vi "Scene info analyzer.vi"(6 "Map Entity Object Position":T2(array[cluster]), 7 "Current Player ID":i32, 8 "Max Player ID":i32) -> (0 "Enemy on 8 directions":T3, 1 "Closest valid target":T1, 2 "Farther Bullets on 8 directions":T3, 3 "Closer Bullets on 8 directions":T3, 4 "Current Player HP":dbl, 5 "Object on 8 directions":T3)   [LabVIEW 2021]
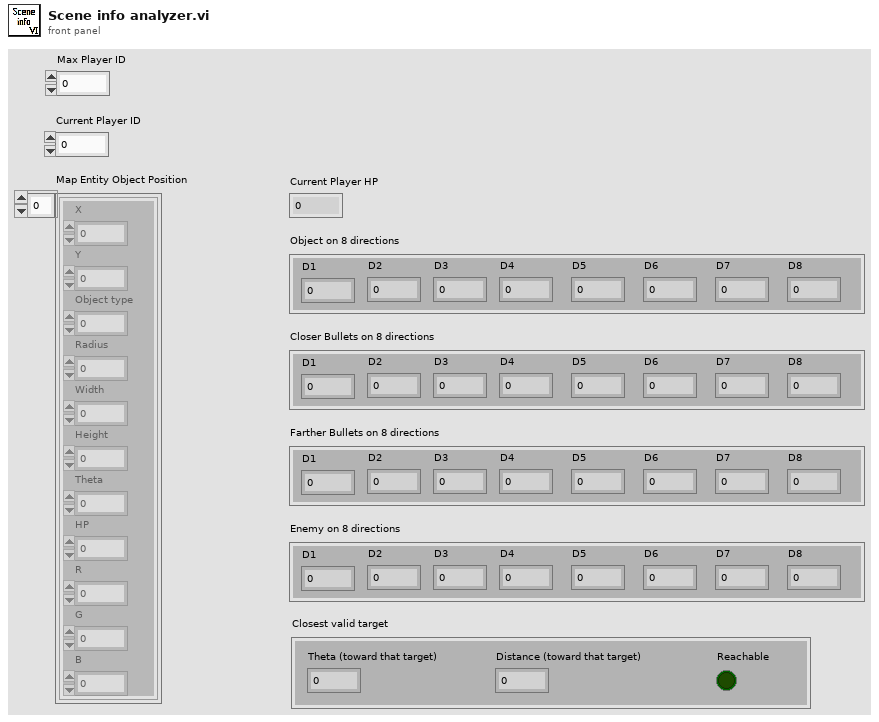
[diagram p1: front panel]
types:
  T1 = cluster{"Theta (toward that target)":dbl, "Distance (toward that target)":dbl, "Reachable":bool}
  T2 = cluster{"X":dbl, "Y":dbl, "Object type":dbl, "Radius":dbl, "Width":dbl, "Height":dbl, "Theta":dbl, "HP":dbl, "R":dbl, "G":dbl, "B":dbl}[]
  T3 = cluster{"D1":dbl, "D2":dbl, "D3":dbl, "D4":dbl, "D5":dbl, "D6":dbl, "D7":dbl, "D8":dbl}
  T4 = cluster{"X":dbl, "Y":dbl, "Object type":dbl, "Radius":dbl, "Width":dbl, "Height":dbl, "Theta":dbl, "HP":dbl, "R":dbl, "G":dbl, "B":dbl}
  T5 = cluster{"X":dbl, "Y":dbl, "Theta (toward that target)":dbl, "Theta (toward that target)":dbl, "Theta (toward that target)":dbl, "Theta (toward that target)":dbl}
  T6 = cluster{dbl, dbl, "Theta (toward that target)":dbl, "Theta (toward that target)":dbl, "Theta (toward that target)":dbl, "Theta (toward that target)":dbl}
  T7 = cluster{dbl, "D2":dbl, "D3":dbl, "D4":dbl, "D5":dbl, "D6":dbl, "D7":dbl, "D8":dbl}
  T8 = cluster{"D1":dbl, dbl, "D3":dbl, "D4":dbl, "D5":dbl, "D6":dbl, "D7":dbl, "D8":dbl}
  T9 = cluster{"D1":dbl, "D2":dbl, dbl, "D4":dbl, "D5":dbl, "D6":dbl, "D7":dbl, "D8":dbl}
  T10 = cluster{"D1":dbl, "D2":dbl, "D3":dbl, dbl, "D5":dbl, "D6":dbl, "D7":dbl, "D8":dbl}
  T11 = cluster{"D1":dbl, "D2":dbl, "D3":dbl, "D4":dbl, dbl, "D6":dbl, "D7":dbl, "D8":dbl}
  T12 = cluster{"D1":dbl, "D2":dbl, "D3":dbl, "D4":dbl, "D5":dbl, dbl, "D7":dbl, "D8":dbl}
  T13 = cluster{"D1":dbl, "D2":dbl, "D3":dbl, "D4":dbl, "D5":dbl, "D6":dbl, dbl, "D8":dbl}
  T14 = cluster{"D1":dbl, "D2":dbl, "D3":dbl, "D4":dbl, "D5":dbl, "D6":dbl, "D7":dbl, dbl}
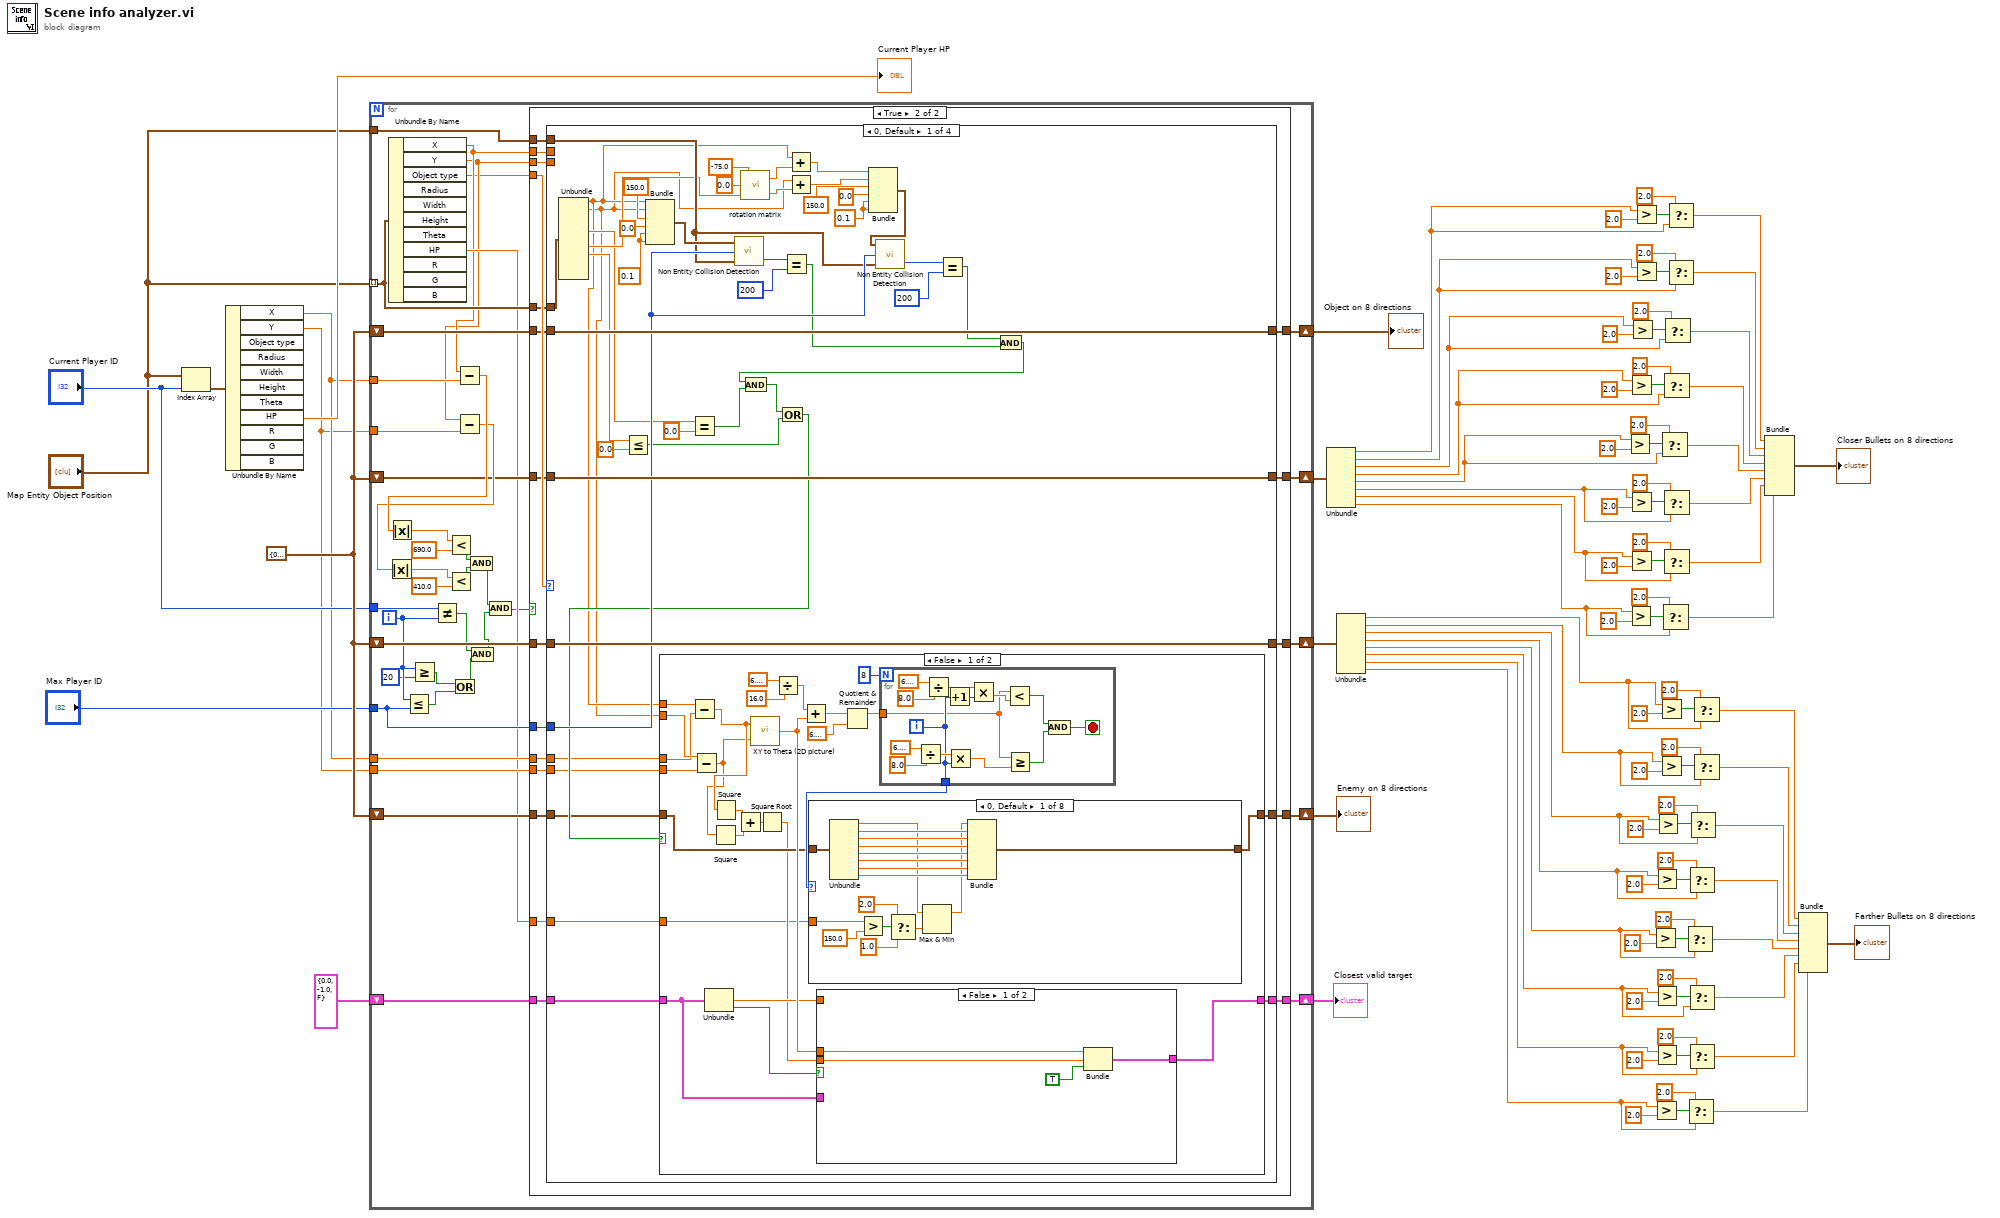
[diagram p0: block diagram]
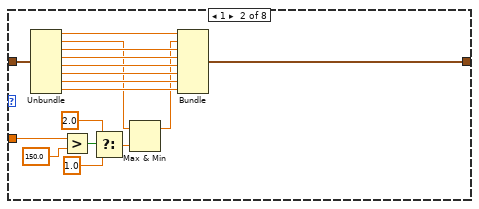
[diagram p3: hidden frame]
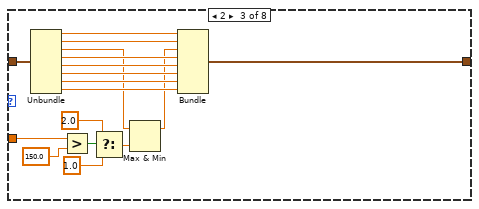
[diagram p4: hidden frame]
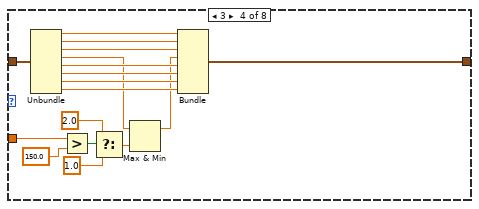
[diagram p5: hidden frame]
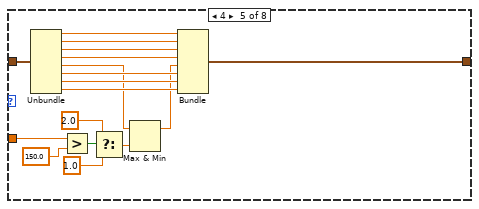
[diagram p6: hidden frame]
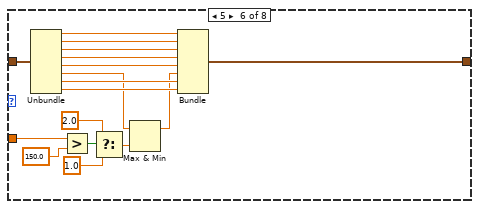
[diagram p7: hidden frame]
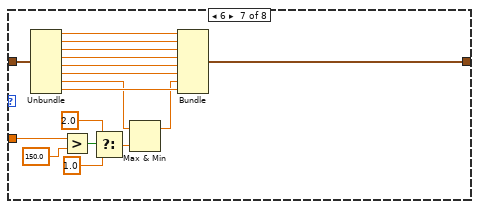
[diagram p8: hidden frame]
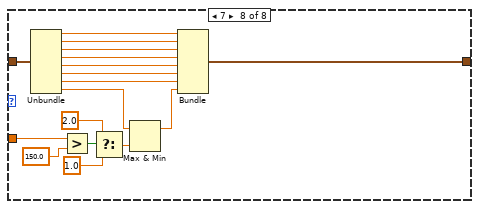
[diagram p9: hidden frame]
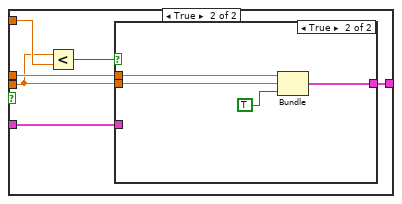
[diagram p10: hidden frame]
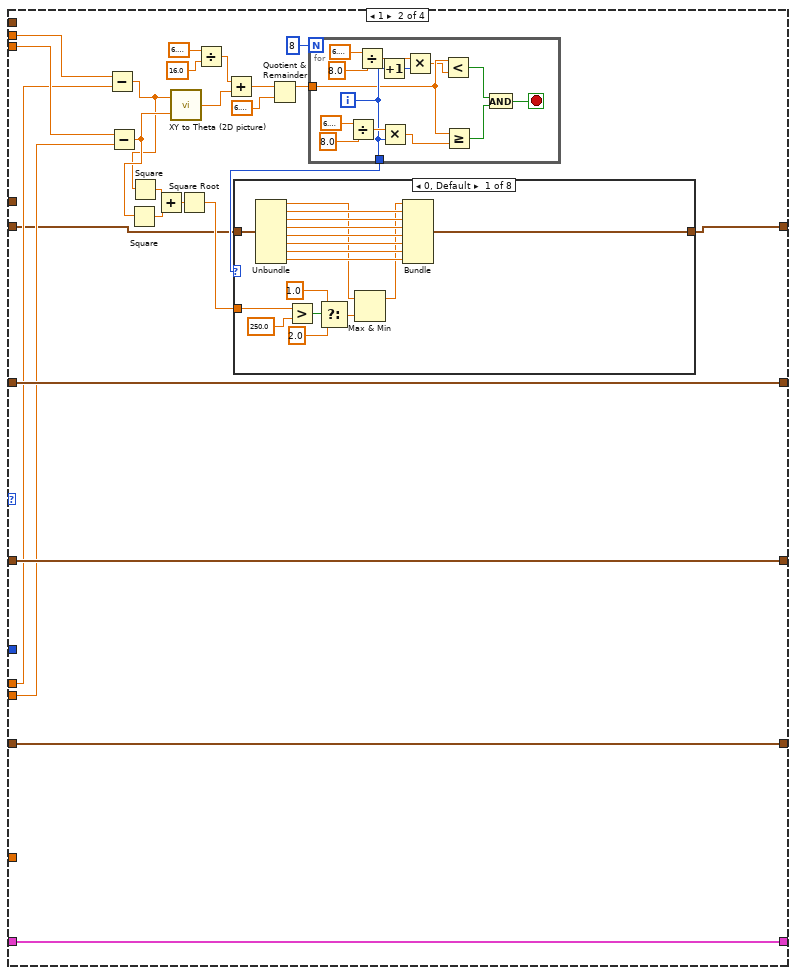
[diagram p13: hidden frame]
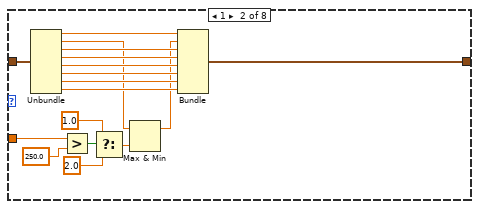
[diagram p14: hidden frame]
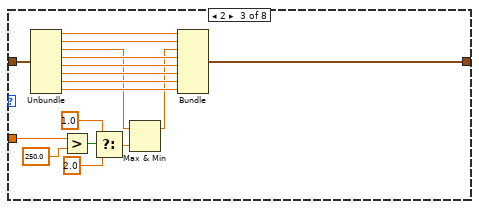
[diagram p15: hidden frame]
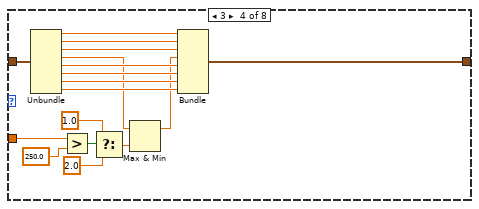
[diagram p16: hidden frame]
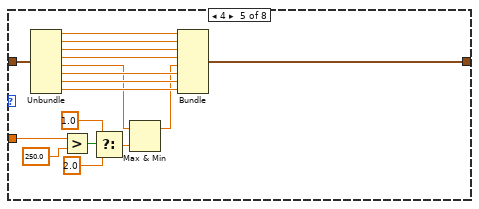
[diagram p17: hidden frame]
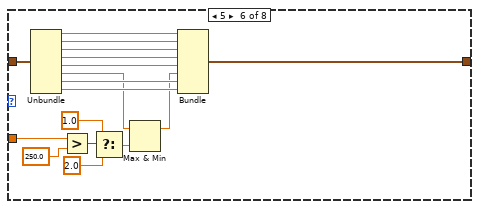
[diagram p18: hidden frame]
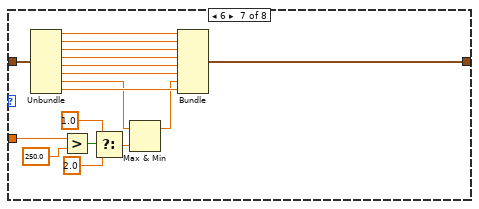
[diagram p19: hidden frame]
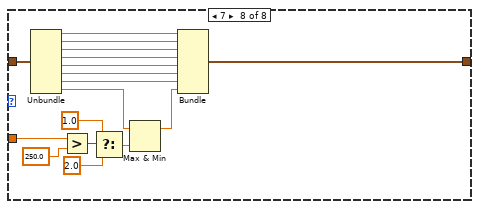
[diagram p20: hidden frame]
diagram:
  w93 = T3 {"D1"=0.0, "D2"=0.0, "D3"=0.0, "D4"=0.0, "D5"=0.0, "D6"=0.0, "D7"=0.0, "D8"=0.0} ("Object on 8 directions")
  n1 = Index Array(array="Map Entity Object Position", index="Current Player ID") -> (element=w96:T4)
  n2 = Unbundle By Name(w96) -> ("X"=w86:dbl, "Y"=w85:dbl, "HP"=→"Current Player HP":dbl)  [unwired: 8 out]
  n3 = for {
    shift-right: [w124] -> w94
    shift-left: w93 -> [w123]
    shift-right: [w122] -> w81
    shift-left: w93 -> [w121]
    shift-right: [w120] -> w80
    shift-left: w93 -> [w119]
    shift-right: [w117] -> w92
    shift-left: w93 -> [w118]
    tunnel: "Map Entity Object Position" -> [w110] mode=indexing
    tunnel: "Current Player ID" -> [w99]
    tunnel: w86 -> [w130]
    tunnel: w85 -> [w129]
    shift-right: [w115] -> w89
    shift-left: T1 {"Theta (toward that target)"=0.0, "Distance (toward that target)"=-1.0, "Reachable"=FALSE} ("Closest valid target") -> [w116]
    tunnel: "Max Player ID" -> [w108]
    tunnel: "Map Entity Object Position" -> [w109]
    tunnel: w86 -> [w107]
    tunnel: w85 -> [w106]
    i -> [w112]
    n4 = Unbundle By Name(w110) -> ("X"=w104:dbl, "Y"=w103:dbl, "Object type"=w98:dbl, "HP"=w105:dbl)  [unwired: 7 out]
    n5 = Less Or Equal?(x=w112, y=w108) -> (x <= y?=w114:bool)
    n6 = Greater Or Equal?(x=w112, y=20) -> (x >= y?=w113:bool)
    n7 = Not Equal?(x=w99, y=w112) -> (x != y?=w100:bool)
    n8 = Or(x=w113, y=w114) -> (x .or. y?=w102:bool)
    n9 = Subtract(x=w104, y=w130) -> (x-y=w126:dbl)
    n10 = Absolute Value(x=w126) -> (abs(x)=w128:dbl)
    n11 = Less?(x=w128, y=690.0) -> (x < y?=w134:bool)
    n12 = Subtract(x=w103, y=w129) -> (x-y=w125:dbl)
    n13 = Absolute Value(x=w125) -> (abs(x)=w127:dbl)
    n14 = Less?(x=w127, y=410.0) -> (x < y?=w133:bool)
    n15 = And(x=w134, y=w133) -> (x .and. y?=w135:bool)
    n16 = And(x=w100, y=w102) -> (x .and. y?=w101:bool)
    n17 = And(x=w135, y=w101) -> (x .and. y?=w97:bool)
    n18 = case shown="True" w97 {
      tunnel: [w140 w158] -> w124
      tunnel: w123 -> [w140 w157]
      tunnel: [w139 w156] -> w122
      tunnel: w121 -> [w139 w155]
      tunnel: [w138 w154] -> w120
      tunnel: w119 -> [w138 w153]
      tunnel: [w137 w149] -> w117
      tunnel: w118 -> [w137 w148]
      tunnel: [w136 w147] -> w115
      tunnel: w116 -> [w136 w146]
      tunnel: w98 -> [_ w159]
      tunnel: w110 -> [_ w152]
      tunnel: w109 -> [_ w151]
      tunnel: w108 -> [_ w150]
      tunnel: w107 -> [_ w145]
      tunnel: w106 -> [_ w144]
      tunnel: w105 -> [_ w143]
      tunnel: w104 -> [_ w142]
      tunnel: w103 -> [_ w141]
      frame False {
      }
      frame True {
        n19 = case shown="0, Default" w159 {
          tunnel: [w204 w398 w573 w752] -> w158
          tunnel: w157 -> [w204 w399 w574 w752]
          tunnel: [w203 w422 w597 w748] -> w156
          tunnel: w155 -> [w203 w422 w597 w751]
          tunnel: [w202 w421 w596 w749] -> w154
          tunnel: w153 -> [w202 w421 w596 w750]
          tunnel: w152 -> [w201 _ _ _]
          tunnel: w151 -> [w190 _ _ _]
          tunnel: w150 -> [w191 _ _ _]
          tunnel: [w173 w420 w595 w773] -> w149
          tunnel: w148 -> [w172 w420 w595 w773]
          tunnel: [w171 w419 w594 w772] -> w147
          tunnel: w146 -> [w170 w419 w594 w772]
          tunnel: w145 -> [w166 w401 w576 w754]
          tunnel: w144 -> [w165 w400 w575 w753]
          tunnel: w143 -> [w164 _ _ _]
          tunnel: w142 -> [_ w403 w578 w756]
          tunnel: w141 -> [_ w402 w577 w755]
          frame 0, Default {
            w193 = 0.1 ("Theta (toward that target)")
            w198 = 0.1 ("Theta (toward that target)")
            n20 = Unbundle(w201) -> ("X"=w168:dbl, "Y"=w167:dbl, "Width"=w177:dbl, "Theta"=w187:dbl, "HP"=w179:dbl)  [unwired: 6 out]
            n21 = Less Or Equal?(x=w179, y=0.0) -> (x <= y?=w169:bool)
            n22 = Bundle("X"=w168, "Y"=w167, "Theta (toward that target)"=150.0, "Theta (toward that target)"=0.0, "Theta (toward that target)"=w198, "Theta (toward that target)"=w198) -> (w197:T5)  [unwired: 1 in]
            n23 = Equal?(x=w177, y=0.0) -> (x = y?=w160:bool)
            n24 = call "Non Entity Collision Detection.vi"("Map Entity Objects Positions"=w190, "Max Player ID number"=w191, "Moving Object"=w197) -> ("Bullet hit Player No."=w196:i32)  [unwired: 1 out]
            n25 = call "rotation matrix.vi"("angle"=w187, "y"=0.0, "x"=-75.0) -> ("new y"=w180:dbl, "new x"=w181:dbl)
            n26 = Equal?(x=w196, y=200) -> (x = y?=w161:bool)
            n27 = Add(x=w168, y=w181) -> (x+y=w182:dbl)
            n28 = Add(x=w167, y=w180) -> (x+y=w183:dbl)
            n29 = Bundle(w182, w183, "Theta (toward that target)"=150.0, "Theta (toward that target)"=0.0, "Theta (toward that target)"=w193, "Theta (toward that target)"=w193) -> (w184:T6)  [unwired: 1 in]
            n30 = call "Non Entity Collision Detection.vi"("Map Entity Objects Positions"=w190, "Max Player ID number"=w191, "Moving Object"=w184) -> ("Bullet hit Player No."=w185:i32)  [unwired: 1 out]
            n31 = Equal?(x=w185, y=200) -> (x = y?=w162:bool)
            n32 = And(x=w162, y=w161) -> (x .and. y?=w163:bool)
            n33 = And(x=w163, y=w160) -> (x .and. y?=w175:bool)
            n34 = Or(x=w175, y=w169) -> (x .or. y?=w174:bool)
            n35 = case shown="False" w174 {
              tunnel: [w207 w397] -> w173
              tunnel: w172 -> [w208 w397]
              tunnel: [w218 w396] -> w171
              tunnel: w170 -> [w210 w396]
              tunnel: w168 -> [w230 _]
              tunnel: w167 -> [w229 _]
              tunnel: w166 -> [w227 _]
              tunnel: w165 -> [w228 _]
              tunnel: w164 -> [w205 _]
              frame False {
                n36 = Subtract(x=w230, y=w227) -> (x-y=w213:dbl)
                n37 = Subtract(x=w229, y=w228) -> (x-y=w212:dbl)
                n38 = Unbundle(w210) -> ("Distance (toward that target)"=w211:dbl, "Reachable"=w219:bool)  [unwired: 1 out]
                n39 = Square(x=w212) -> (x^2=w215:dbl)
                n40 = Square(x=w213) -> (x^2=w216:dbl)
                n41 = Add(x=w216, y=w215) -> (x+y=w214:dbl)
                n42 = call "XY to Theta (2D picture).vi"("y"=w212, "x"=w213) -> ("Theta"=w217:dbl)
                n43 = Square Root(x=w214) -> (sqrt(x)=w206:dbl)
                n44 = Divide(x=6.283185307179586, y=16.0) -> (x/y=w224:dbl)
                n45 = Add(x=w224, y=w217) -> (x+y=w223:dbl)
                n46 = case shown="False" w219 {
                  tunnel: [w369 w374] -> w218
                  tunnel: w217 -> [w368 w372]
                  tunnel: w206 -> [w367 w371]
                  tunnel: w211 -> [_ w376]
                  tunnel: w210 -> [_ w373]
                  frame False {
                    n47 = Bundle("Theta"=w368, w367, "Reachable"=TRUE) -> (w369:cluster{"Theta":dbl, dbl, "Reachable":bool})  [unwired: 1 in]
                  }
                  frame True {
                    n48 = Less?(x=w371, y=w376) -> (x < y?=w375:bool)
                    n49 = case shown="True" w375 {
                      tunnel: [w377 w380] -> w374
                      tunnel: w373 -> [w377 _]
                      tunnel: w372 -> [_ w379]
                      tunnel: w371 -> [_ w378]
                      frame False {
                      }
                      frame True {
                        n50 = Bundle("Theta"=w379, w378, "Reachable"=TRUE) -> (w380:cluster{"Theta":dbl, dbl, "Reachable":bool})  [unwired: 1 in]
                      }
                    }
                  }
                }
                n51 = Quotient & Remainder(x=w223, y=6.283185307179586) -> (x-y*floor(x/y)=w221:dbl)  [unwired: 1 out]
                n52 = for {
                  N: 8 -> [_]
                  tunnel: w221 -> [w383]
                  tunnel: [w385] -> w209
                  i -> [w385]
                  stop <- w386 stop-if-true
                  n53 = Divide(x=6.283185307179586, y=8.0) -> (x/y=w393:dbl)
                  n54 = Divide(x=6.283185307179586, y=8.0) -> (x/y=w390:dbl)
                  n55 = Increment(x=w385) -> (x+1=w389:i32)
                  n56 = Multiply(x=w393, y=w385) -> (x*y=w382:dbl)
                  n57 = Multiply(x=w390, y=w389) -> (x*y=w384:dbl)
                  n58 = Less?(x=w383, y=w384) -> (x < y?=w388:bool)
                  n59 = Greater Or Equal?(x=w383, y=w382) -> (x >= y?=w387:bool)
                  n60 = And(x=w388, y=w387) -> (x .and. y?=w386:bool)
                }
                n61 = case shown="0, Default" w209 {
                  tunnel: w208 -> [w247 w264 w281 w298 w315 w332 w349 w366]
                  tunnel: [w231 w251 w269 w287 w305 w323 w341 w359] -> w207
                  tunnel: w205 -> [w237 w255 w273 w291 w309 w327 w345 w363]
                  frame 0, Default {
                    n62 = Unbundle(w247) -> ("D1"=w233:dbl, "D2"=w244:dbl, "D3"=w243:dbl, "D4"=w242:dbl, "D5"=w241:dbl, "D6"=w240:dbl, "D7"=w239:dbl, "D8"=w238:dbl)
                    n63 = Greater?(x=w237, y=150.0) -> (0:w246:bool)
                    n64 = Select(t=2.0, s=w246, f=1.0) -> (s? t:f=w234:dbl)
                    n65 = Max & Min(x=w233, y=w234) -> (max(x,y)=w232:dbl)  [unwired: 1 out]
                    n66 = Bundle(w232, "D2"=w244, "D3"=w243, "D4"=w242, "D5"=w241, "D6"=w240, "D7"=w239, "D8"=w238) -> (w231:T7)  [unwired: 1 in]
                  }
                  frame 1 {
                    n67 = Unbundle(w264) -> ("D1"=w250:dbl, "D2"=w249:dbl, "D3"=w261:dbl, "D4"=w260:dbl, "D5"=w259:dbl, "D6"=w258:dbl, "D7"=w257:dbl, "D8"=w256:dbl)
                    n68 = Greater?(x=w255, y=150.0) -> (0:w263:bool)
                    n69 = Select(t=2.0, s=w263, f=1.0) -> (s? t:f=w252:dbl)
                    n70 = Max & Min(x=w249, y=w252) -> (max(x,y)=w248:dbl)  [unwired: 1 out]
                    n71 = Bundle("D1"=w250, w248, "D3"=w261, "D4"=w260, "D5"=w259, "D6"=w258, "D7"=w257, "D8"=w256) -> (w251:T8)  [unwired: 1 in]
                  }
                  frame 2 {
                    n72 = Unbundle(w281) -> ("D1"=w268:dbl, "D2"=w267:dbl, "D3"=w266:dbl, "D4"=w278:dbl, "D5"=w277:dbl, "D6"=w276:dbl, "D7"=w275:dbl, "D8"=w274:dbl)
                    n73 = Greater?(x=w273, y=150.0) -> (0:w280:bool)
                    n74 = Select(t=2.0, s=w280, f=1.0) -> (s? t:f=w270:dbl)
                    n75 = Max & Min(x=w266, y=w270) -> (max(x,y)=w265:dbl)  [unwired: 1 out]
                    n76 = Bundle("D1"=w268, "D2"=w267, w265, "D4"=w278, "D5"=w277, "D6"=w276, "D7"=w275, "D8"=w274) -> (w269:T9)  [unwired: 1 in]
                  }
                  frame 3 {
                    n77 = Unbundle(w298) -> ("D1"=w286:dbl, "D2"=w285:dbl, "D3"=w284:dbl, "D4"=w283:dbl, "D5"=w295:dbl, "D6"=w294:dbl, "D7"=w293:dbl, "D8"=w292:dbl)
                    n78 = Greater?(x=w291, y=150.0) -> (0:w297:bool)
                    n79 = Select(t=2.0, s=w297, f=1.0) -> (s? t:f=w288:dbl)
                    n80 = Max & Min(x=w283, y=w288) -> (max(x,y)=w282:dbl)  [unwired: 1 out]
                    n81 = Bundle("D1"=w286, "D2"=w285, "D3"=w284, w282, "D5"=w295, "D6"=w294, "D7"=w293, "D8"=w292) -> (w287:T10)  [unwired: 1 in]
                  }
                  frame 4 {
                    n82 = Unbundle(w315) -> ("D1"=w304:dbl, "D2"=w303:dbl, "D3"=w302:dbl, "D4"=w299:dbl, "D5"=w301:dbl, "D6"=w312:dbl, "D7"=w311:dbl, "D8"=w310:dbl)
                    n83 = Greater?(x=w309, y=150.0) -> (0:w314:bool)
                    n84 = Select(t=2.0, s=w314, f=1.0) -> (s? t:f=w306:dbl)
                    n85 = Max & Min(x=w301, y=w306) -> (max(x,y)=w300:dbl)  [unwired: 1 out]
                    n86 = Bundle("D1"=w304, "D2"=w303, "D3"=w302, "D4"=w299, w300, "D6"=w312, "D7"=w311, "D8"=w310) -> (w305:T11)  [unwired: 1 in]
                  }
                  frame 5 {
                    n87 = Unbundle(w332) -> ("D1"=w322:dbl, "D2"=w321:dbl, "D3"=w320:dbl, "D4"=w319:dbl, "D5"=w318:dbl, "D6"=w317:dbl, "D7"=w329:dbl, "D8"=w328:dbl)
                    n88 = Greater?(x=w327, y=150.0) -> (0:w331:bool)
                    n89 = Select(t=2.0, s=w331, f=1.0) -> (s? t:f=w324:dbl)
                    n90 = Max & Min(x=w317, y=w324) -> (max(x,y)=w316:dbl)  [unwired: 1 out]
                    n91 = Bundle("D1"=w322, "D2"=w321, "D3"=w320, "D4"=w319, "D5"=w318, w316, "D7"=w329, "D8"=w328) -> (w323:T12)  [unwired: 1 in]
                  }
                  frame 6 {
                    n92 = Unbundle(w349) -> ("D1"=w340:dbl, "D2"=w339:dbl, "D3"=w338:dbl, "D4"=w337:dbl, "D5"=w336:dbl, "D6"=w333:dbl, "D7"=w335:dbl, "D8"=w346:dbl)
                    n93 = Greater?(x=w345, y=150.0) -> (0:w348:bool)
                    n94 = Select(t=2.0, s=w348, f=1.0) -> (s? t:f=w342:dbl)
                    n95 = Max & Min(x=w335, y=w342) -> (max(x,y)=w334:dbl)  [unwired: 1 out]
                    n96 = Bundle("D1"=w340, "D2"=w339, "D3"=w338, "D4"=w337, "D5"=w336, "D6"=w333, w334, "D8"=w346) -> (w341:T13)  [unwired: 1 in]
                  }
                  frame 7 {
                    n97 = Unbundle(w366) -> ("D1"=w358:dbl, "D2"=w357:dbl, "D3"=w356:dbl, "D4"=w355:dbl, "D5"=w354:dbl, "D6"=w353:dbl, "D7"=w352:dbl, "D8"=w351:dbl)
                    n98 = Greater?(x=w363, y=150.0) -> (0:w365:bool)
                    n99 = Select(t=2.0, s=w365, f=1.0) -> (s? t:f=w360:dbl)
                    n100 = Max & Min(x=w351, y=w360) -> (max(x,y)=w350:dbl)  [unwired: 1 out]
                    n101 = Bundle("D1"=w358, "D2"=w357, "D3"=w356, "D4"=w355, "D5"=w354, "D6"=w353, "D7"=w352, w350) -> (w359:T14)  [unwired: 1 in]
                  }
                }
              }
              frame True {
              }
            }
          }
          frame 1 {
            n102 = Subtract(x=w403, y=w401) -> (x-y=w415:dbl)
            n103 = Subtract(x=w402, y=w400) -> (x-y=w416:dbl)
            n104 = Square(x=w416) -> (x^2=w413:dbl)
            n105 = Square(x=w415) -> (x^2=w412:dbl)
            n106 = Add(x=w412, y=w413) -> (x+y=w414:dbl)
            n107 = call "XY to Theta (2D picture).vi"("y"=w416, "x"=w415) -> ("Theta"=w411:dbl)
            n108 = Square Root(x=w414) -> (sqrt(x)=w418:dbl)
            n109 = Divide(x=6.283185307179586, y=16.0) -> (x/y=w408:dbl)
            n110 = Add(x=w408, y=w411) -> (x+y=w409:dbl)
            n111 = Quotient & Remainder(x=w409, y=6.283185307179586) -> (x-y*floor(x/y)=w410:dbl)  [unwired: 1 out]
            n112 = for {
              N: 8 -> [_]
              tunnel: w410 -> [w561]
              tunnel: [w562] -> w417
              i -> [w562]
              stop <- w563 stop-if-true
              n113 = Divide(x=6.283185307179586, y=8.0) -> (x/y=w570:dbl)
              n114 = Divide(x=6.283185307179586, y=8.0) -> (x/y=w567:dbl)
              n115 = Increment(x=w562) -> (x+1=w566:i32)
              n116 = Multiply(x=w570, y=w562) -> (x*y=w559:dbl)
              n117 = Multiply(x=w567, y=w566) -> (x*y=w560:dbl)
              n118 = Less?(x=w561, y=w560) -> (x < y?=w565:bool)
              n119 = Greater Or Equal?(x=w561, y=w559) -> (x >= y?=w564:bool)
              n120 = And(x=w565, y=w564) -> (x .and. y?=w563:bool)
            }
            n121 = case shown="0, Default" w417 {
              tunnel: w399 -> [w439 w456 w473 w490 w507 w524 w541 w558]
              tunnel: [w423 w443 w461 w479 w497 w515 w533 w551] -> w398
              tunnel: w418 -> [w429 w447 w465 w483 w501 w519 w537 w555]
              frame 0, Default {
                n122 = Unbundle(w439) -> ("D1"=w425:dbl, "D2"=w436:dbl, "D3"=w435:dbl, "D4"=w434:dbl, "D5"=w433:dbl, "D6"=w432:dbl, "D7"=w431:dbl, "D8"=w430:dbl)
                n123 = Greater?(x=w429, y=250.0) -> (0:w438:bool)
                n124 = Select(t=1.0, s=w438, f=2.0) -> (s? t:f=w426:dbl)
                n125 = Max & Min(x=w425, y=w426) -> (max(x,y)=w424:dbl)  [unwired: 1 out]
                n126 = Bundle(w424, "D2"=w436, "D3"=w435, "D4"=w434, "D5"=w433, "D6"=w432, "D7"=w431, "D8"=w430) -> (w423:T7)  [unwired: 1 in]
              }
              frame 1 {
                n127 = Unbundle(w456) -> ("D1"=w442:dbl, "D2"=w441:dbl, "D3"=w453:dbl, "D4"=w452:dbl, "D5"=w451:dbl, "D6"=w450:dbl, "D7"=w449:dbl, "D8"=w448:dbl)
                n128 = Greater?(x=w447, y=250.0) -> (0:w455:bool)
                n129 = Select(t=1.0, s=w455, f=2.0) -> (s? t:f=w444:dbl)
                n130 = Max & Min(x=w441, y=w444) -> (max(x,y)=w440:dbl)  [unwired: 1 out]
                n131 = Bundle("D1"=w442, w440, "D3"=w453, "D4"=w452, "D5"=w451, "D6"=w450, "D7"=w449, "D8"=w448) -> (w443:T8)  [unwired: 1 in]
              }
              frame 2 {
                n132 = Unbundle(w473) -> ("D1"=w460:dbl, "D2"=w459:dbl, "D3"=w458:dbl, "D4"=w470:dbl, "D5"=w469:dbl, "D6"=w468:dbl, "D7"=w467:dbl, "D8"=w466:dbl)
                n133 = Greater?(x=w465, y=250.0) -> (0:w472:bool)
                n134 = Select(t=1.0, s=w472, f=2.0) -> (s? t:f=w462:dbl)
                n135 = Max & Min(x=w458, y=w462) -> (max(x,y)=w457:dbl)  [unwired: 1 out]
                n136 = Bundle("D1"=w460, "D2"=w459, w457, "D4"=w470, "D5"=w469, "D6"=w468, "D7"=w467, "D8"=w466) -> (w461:T9)  [unwired: 1 in]
              }
              frame 3 {
                n137 = Unbundle(w490) -> ("D1"=w478:dbl, "D2"=w477:dbl, "D3"=w476:dbl, "D4"=w475:dbl, "D5"=w487:dbl, "D6"=w486:dbl, "D7"=w485:dbl, "D8"=w484:dbl)
                n138 = Greater?(x=w483, y=250.0) -> (0:w489:bool)
                n139 = Select(t=1.0, s=w489, f=2.0) -> (s? t:f=w480:dbl)
                n140 = Max & Min(x=w475, y=w480) -> (max(x,y)=w474:dbl)  [unwired: 1 out]
                n141 = Bundle("D1"=w478, "D2"=w477, "D3"=w476, w474, "D5"=w487, "D6"=w486, "D7"=w485, "D8"=w484) -> (w479:T10)  [unwired: 1 in]
              }
              frame 4 {
                n142 = Unbundle(w507) -> ("D1"=w496:dbl, "D2"=w495:dbl, "D3"=w494:dbl, "D4"=w491:dbl, "D5"=w493:dbl, "D6"=w504:dbl, "D7"=w503:dbl, "D8"=w502:dbl)
                n143 = Greater?(x=w501, y=250.0) -> (0:w506:bool)
                n144 = Select(t=1.0, s=w506, f=2.0) -> (s? t:f=w498:dbl)
                n145 = Max & Min(x=w493, y=w498) -> (max(x,y)=w492:dbl)  [unwired: 1 out]
                n146 = Bundle("D1"=w496, "D2"=w495, "D3"=w494, "D4"=w491, w492, "D6"=w504, "D7"=w503, "D8"=w502) -> (w497:T11)  [unwired: 1 in]
              }
              frame 5 {
                n147 = Unbundle(w524) -> ("D1"=w514:dbl, "D2"=w513:dbl, "D3"=w512:dbl, "D4"=w511:dbl, "D5"=w510:dbl, "D6"=w509:dbl, "D7"=w521:dbl, "D8"=w520:dbl)
                n148 = Greater?(x=w519, y=250.0) -> (0:w523:bool)
                n149 = Select(t=1.0, s=w523, f=2.0) -> (s? t:f=w516:dbl)
                n150 = Max & Min(x=w509, y=w516) -> (max(x,y)=w508:dbl)  [unwired: 1 out]
                n151 = Bundle("D1"=w514, "D2"=w513, "D3"=w512, "D4"=w511, "D5"=w510, w508, "D7"=w521, "D8"=w520) -> (w515:T12)  [unwired: 1 in]
              }
              frame 6 {
                n152 = Unbundle(w541) -> ("D1"=w532:dbl, "D2"=w531:dbl, "D3"=w530:dbl, "D4"=w529:dbl, "D5"=w528:dbl, "D6"=w525:dbl, "D7"=w527:dbl, "D8"=w538:dbl)
                n153 = Greater?(x=w537, y=250.0) -> (0:w540:bool)
                n154 = Select(t=1.0, s=w540, f=2.0) -> (s? t:f=w534:dbl)
                n155 = Max & Min(x=w527, y=w534) -> (max(x,y)=w526:dbl)  [unwired: 1 out]
                n156 = Bundle("D1"=w532, "D2"=w531, "D3"=w530, "D4"=w529, "D5"=w528, "D6"=w525, w526, "D8"=w538) -> (w533:T13)  [unwired: 1 in]
              }
              frame 7 {
                n157 = Unbundle(w558) -> ("D1"=w550:dbl, "D2"=w549:dbl, "D3"=w548:dbl, "D4"=w547:dbl, "D5"=w546:dbl, "D6"=w545:dbl, "D7"=w544:dbl, "D8"=w543:dbl)
                n158 = Greater?(x=w555, y=250.0) -> (0:w557:bool)
                n159 = Select(t=1.0, s=w557, f=2.0) -> (s? t:f=w552:dbl)
                n160 = Max & Min(x=w543, y=w552) -> (max(x,y)=w542:dbl)  [unwired: 1 out]
                n161 = Bundle("D1"=w550, "D2"=w549, "D3"=w548, "D4"=w547, "D5"=w546, "D6"=w545, "D7"=w544, w542) -> (w551:T14)  [unwired: 1 in]
              }
            }
          }
          frame 2 {
            n162 = Subtract(x=w578, y=w576) -> (x-y=w590:dbl)
            n163 = Subtract(x=w577, y=w575) -> (x-y=w591:dbl)
            n164 = Square(x=w591) -> (x^2=w588:dbl)
            n165 = Square(x=w590) -> (x^2=w587:dbl)
            n166 = Add(x=w587, y=w588) -> (x+y=w589:dbl)
            n167 = call "XY to Theta (2D picture).vi"("y"=w591, "x"=w590) -> ("Theta"=w586:dbl)
            n168 = Square Root(x=w589) -> (sqrt(x)=w593:dbl)
            n169 = Divide(x=6.283185307179586, y=16.0) -> (x/y=w583:dbl)
            n170 = Add(x=w583, y=w586) -> (x+y=w584:dbl)
            n171 = Quotient & Remainder(x=w584, y=6.283185307179586) -> (x-y*floor(x/y)=w585:dbl)  [unwired: 1 out]
            n172 = for {
              N: 8 -> [_]
              tunnel: w585 -> [w735]
              tunnel: [w737] -> w592
              i -> [w737]
              stop <- w738 stop-if-true
              n173 = Divide(x=6.283185307179586, y=8.0) -> (x/y=w745:dbl)
              n174 = Divide(x=6.283185307179586, y=8.0) -> (x/y=w742:dbl)
              n175 = Increment(x=w737) -> (x+1=w741:i32)
              n176 = Multiply(x=w745, y=w737) -> (x*y=w736:dbl)
              n177 = Multiply(x=w742, y=w741) -> (x*y=w734:dbl)
              n178 = Less?(x=w735, y=w734) -> (x < y?=w740:bool)
              n179 = Greater Or Equal?(x=w735, y=w736) -> (x >= y?=w739:bool)
              n180 = And(x=w740, y=w739) -> (x .and. y?=w738:bool)
            }
            n181 = case shown="0, Default" w592 {
              tunnel: w574 -> [w614 w631 w648 w665 w682 w699 w716 w733]
              tunnel: [w598 w618 w636 w654 w672 w690 w708 w726] -> w573
              tunnel: w593 -> [w604 w622 w640 w658 w676 w694 w712 w730]
              frame 0, Default {
                n182 = Unbundle(w614) -> ("D1"=w600:dbl, "D2"=w611:dbl, "D3"=w610:dbl, "D4"=w609:dbl, "D5"=w608:dbl, "D6"=w607:dbl, "D7"=w606:dbl, "D8"=w605:dbl)
                n183 = Greater?(x=w604, y=250.0) -> (0:w613:bool)
                n184 = Select(t=1.0, s=w613, f=2.0) -> (s? t:f=w601:dbl)
                n185 = Max & Min(x=w600, y=w601) -> (max(x,y)=w599:dbl)  [unwired: 1 out]
                n186 = Bundle(w599, "D2"=w611, "D3"=w610, "D4"=w609, "D5"=w608, "D6"=w607, "D7"=w606, "D8"=w605) -> (w598:T7)  [unwired: 1 in]
              }
              frame 1 {
                n187 = Unbundle(w631) -> ("D1"=w617:dbl, "D2"=w616:dbl, "D3"=w628:dbl, "D4"=w627:dbl, "D5"=w626:dbl, "D6"=w625:dbl, "D7"=w624:dbl, "D8"=w623:dbl)
                n188 = Greater?(x=w622, y=250.0) -> (0:w630:bool)
                n189 = Select(t=1.0, s=w630, f=2.0) -> (s? t:f=w619:dbl)
                n190 = Max & Min(x=w616, y=w619) -> (max(x,y)=w615:dbl)  [unwired: 1 out]
                n191 = Bundle("D1"=w617, w615, "D3"=w628, "D4"=w627, "D5"=w626, "D6"=w625, "D7"=w624, "D8"=w623) -> (w618:T8)  [unwired: 1 in]
              }
              frame 2 {
                n192 = Unbundle(w648) -> ("D1"=w635:dbl, "D2"=w634:dbl, "D3"=w633:dbl, "D4"=w645:dbl, "D5"=w644:dbl, "D6"=w643:dbl, "D7"=w642:dbl, "D8"=w641:dbl)
                n193 = Greater?(x=w640, y=250.0) -> (0:w647:bool)
                n194 = Select(t=1.0, s=w647, f=2.0) -> (s? t:f=w637:dbl)
                n195 = Max & Min(x=w633, y=w637) -> (max(x,y)=w632:dbl)  [unwired: 1 out]
                n196 = Bundle("D1"=w635, "D2"=w634, w632, "D4"=w645, "D5"=w644, "D6"=w643, "D7"=w642, "D8"=w641) -> (w636:T9)  [unwired: 1 in]
              }
              frame 3 {
                n197 = Unbundle(w665) -> ("D1"=w653:dbl, "D2"=w652:dbl, "D3"=w651:dbl, "D4"=w650:dbl, "D5"=w662:dbl, "D6"=w661:dbl, "D7"=w660:dbl, "D8"=w659:dbl)
                n198 = Greater?(x=w658, y=250.0) -> (0:w664:bool)
                n199 = Select(t=1.0, s=w664, f=2.0) -> (s? t:f=w655:dbl)
                n200 = Max & Min(x=w650, y=w655) -> (max(x,y)=w649:dbl)  [unwired: 1 out]
                n201 = Bundle("D1"=w653, "D2"=w652, "D3"=w651, w649, "D5"=w662, "D6"=w661, "D7"=w660, "D8"=w659) -> (w654:T10)  [unwired: 1 in]
              }
              frame 4 {
                n202 = Unbundle(w682) -> ("D1"=w671:dbl, "D2"=w670:dbl, "D3"=w669:dbl, "D4"=w666:dbl, "D5"=w668:dbl, "D6"=w679:dbl, "D7"=w678:dbl, "D8"=w677:dbl)
                n203 = Greater?(x=w676, y=250.0) -> (0:w681:bool)
                n204 = Select(t=1.0, s=w681, f=2.0) -> (s? t:f=w673:dbl)
                n205 = Max & Min(x=w668, y=w673) -> (max(x,y)=w667:dbl)  [unwired: 1 out]
                n206 = Bundle("D1"=w671, "D2"=w670, "D3"=w669, "D4"=w666, w667, "D6"=w679, "D7"=w678, "D8"=w677) -> (w672:T11)  [unwired: 1 in]
              }
              frame 5 {
                n207 = Unbundle(w699) -> ("D1"=w689:dbl, "D2"=w688:dbl, "D3"=w687:dbl, "D4"=w686:dbl, "D5"=w685:dbl, "D6"=w684:dbl, "D7"=w696:dbl, "D8"=w695:dbl)
                n208 = Greater?(x=w694, y=250.0) -> (0:w698:bool)
                n209 = Select(t=1.0, s=w698, f=2.0) -> (s? t:f=w691:dbl)
                n210 = Max & Min(x=w684, y=w691) -> (max(x,y)=w683:dbl)  [unwired: 1 out]
                n211 = Bundle("D1"=w689, "D2"=w688, "D3"=w687, "D4"=w686, "D5"=w685, w683, "D7"=w696, "D8"=w695) -> (w690:T12)  [unwired: 1 in]
              }
              frame 6 {
                n212 = Unbundle(w716) -> ("D1"=w707:dbl, "D2"=w706:dbl, "D3"=w705:dbl, "D4"=w704:dbl, "D5"=w703:dbl, "D6"=w700:dbl, "D7"=w702:dbl, "D8"=w713:dbl)
                n213 = Greater?(x=w712, y=250.0) -> (0:w715:bool)
                n214 = Select(t=1.0, s=w715, f=2.0) -> (s? t:f=w709:dbl)
                n215 = Max & Min(x=w702, y=w709) -> (max(x,y)=w701:dbl)  [unwired: 1 out]
                n216 = Bundle("D1"=w707, "D2"=w706, "D3"=w705, "D4"=w704, "D5"=w703, "D6"=w700, w701, "D8"=w713) -> (w708:T13)  [unwired: 1 in]
              }
              frame 7 {
                n217 = Unbundle(w733) -> ("D1"=w725:dbl, "D2"=w724:dbl, "D3"=w723:dbl, "D4"=w722:dbl, "D5"=w721:dbl, "D6"=w720:dbl, "D7"=w719:dbl, "D8"=w718:dbl)
                n218 = Greater?(x=w730, y=250.0) -> (0:w732:bool)
                n219 = Select(t=1.0, s=w732, f=2.0) -> (s? t:f=w727:dbl)
                n220 = Max & Min(x=w718, y=w727) -> (max(x,y)=w717:dbl)  [unwired: 1 out]
                n221 = Bundle("D1"=w725, "D2"=w724, "D3"=w723, "D4"=w722, "D5"=w721, "D6"=w720, "D7"=w719, w717) -> (w726:T14)  [unwired: 1 in]
              }
            }
          }
          frame 5 {
            n222 = Subtract(x=w756, y=w754) -> (x-y=w768:dbl)
            n223 = Subtract(x=w755, y=w753) -> (x-y=w769:dbl)
            n224 = Square(x=w769) -> (x^2=w766:dbl)
            n225 = Square(x=w768) -> (x^2=w765:dbl)
            n226 = Add(x=w765, y=w766) -> (x+y=w767:dbl)
            n227 = call "XY to Theta (2D picture).vi"("y"=w769, "x"=w768) -> ("Theta"=w764:dbl)
            n228 = Square Root(x=w767) -> (sqrt(x)=w771:dbl)
            n229 = Divide(x=6.283185307179586, y=16.0) -> (x/y=w761:dbl)
            n230 = Add(x=w761, y=w764) -> (x+y=w762:dbl)
            n231 = Quotient & Remainder(x=w762, y=6.283185307179586) -> (x-y*floor(x/y)=w763:dbl)  [unwired: 1 out]
            n232 = for {
              N: 8 -> [_]
              tunnel: w763 -> [w1023]
              tunnel: [w1025] -> w770
              i -> [w1025]
              stop <- w1026 stop-if-true
              n233 = Divide(x=6.283185307179586, y=8.0) -> (x/y=w1033:dbl)
              n234 = Divide(x=6.283185307179586, y=8.0) -> (x/y=w1030:dbl)
              n235 = Increment(x=w1025) -> (x+1=w1029:i32)
              n236 = Multiply(x=w1033, y=w1025) -> (x*y=w1024:dbl)
              n237 = Multiply(x=w1030, y=w1029) -> (x*y=w1022:dbl)
              n238 = Less?(x=w1023, y=w1022) -> (x < y?=w1028:bool)
              n239 = Greater Or Equal?(x=w1023, y=w1024) -> (x >= y?=w1027:bool)
              n240 = And(x=w1028, y=w1027) -> (x .and. y?=w1026:bool)
            }
            n241 = case shown="0, Default" w770 {
              tunnel: w771 -> [w779 w810 w841 w872 w903 w934 w965 w996]
              tunnel: w751 -> [w774 w805 w836 w867 w898 w929 w960 w991]
              tunnel: w750 -> [w777 w808 w839 w870 w901 w932 w963 w994]
              tunnel: [w776 w807 w838 w869 w900 w931 w962 w993] -> w749
              tunnel: [w775 w806 w837 w868 w899 w930 w961 w992] -> w748
              frame 0, Default {
                n242 = Greater?(x=w779, y=250.0) -> (0:w778:bool)
                n243 = case shown="True" w778 {
                  tunnel: w777 -> [w792 w796]
                  tunnel: [w792 w795] -> w776
                  tunnel: [w783 w794] -> w775
                  tunnel: w774 -> [w782 w794]
                  frame False {
                    n244 = Unbundle(w782) -> ("D1"=w784:dbl, "D2"=w791:dbl, "D3"=w790:dbl, "D4"=w789:dbl, "D5"=w788:dbl, "D6"=w787:dbl, "D7"=w786:dbl, "D8"=w785:dbl)
                    n245 = Increment(x=w784) -> (x+1=w781:dbl)
                    n246 = Bundle(w781, "D2"=w791, "D3"=w790, "D4"=w789, "D5"=w788, "D6"=w787, "D7"=w786, "D8"=w785) -> (w783:T7)  [unwired: 1 in]
                  }
                  frame True {
                    n247 = Unbundle(w796) -> ("D1"=w797:dbl, "D2"=w804:dbl, "D3"=w803:dbl, "D4"=w802:dbl, "D5"=w801:dbl, "D6"=w800:dbl, "D7"=w799:dbl, "D8"=w798:dbl)
                    n248 = Increment(x=w797) -> (x+1=w793:dbl)
                    n249 = Bundle(w793, "D2"=w804, "D3"=w803, "D4"=w802, "D5"=w801, "D6"=w800, "D7"=w799, "D8"=w798) -> (w795:T7)  [unwired: 1 in]
                  }
                }
              }
              frame 1 {
                n250 = Greater?(x=w810, y=250.0) -> (0:w809:bool)
                n251 = case shown="True" w809 {
                  tunnel: w808 -> [w823 w828]
                  tunnel: [w823 w827] -> w807
                  tunnel: [w815 w826] -> w806
                  tunnel: w805 -> [w814 w826]
                  frame False {
                    n252 = Unbundle(w814) -> ("D1"=w813:dbl, "D2"=w822:dbl, "D3"=w821:dbl, "D4"=w820:dbl, "D5"=w819:dbl, "D6"=w818:dbl, "D7"=w817:dbl, "D8"=w816:dbl)
                    n253 = Increment(x=w822) -> (x+1=w812:dbl)
                    n254 = Bundle("D1"=w813, w812, "D3"=w821, "D4"=w820, "D5"=w819, "D6"=w818, "D7"=w817, "D8"=w816) -> (w815:T8)  [unwired: 1 in]
                  }
                  frame True {
                    n255 = Unbundle(w828) -> ("D1"=w825:dbl, "D2"=w835:dbl, "D3"=w834:dbl, "D4"=w833:dbl, "D5"=w832:dbl, "D6"=w831:dbl, "D7"=w830:dbl, "D8"=w829:dbl)
                    n256 = Increment(x=w835) -> (x+1=w824:dbl)
                    n257 = Bundle("D1"=w825, w824, "D3"=w834, "D4"=w833, "D5"=w832, "D6"=w831, "D7"=w830, "D8"=w829) -> (w827:T8)  [unwired: 1 in]
                  }
                }
              }
              frame 2 {
                n258 = Greater?(x=w841, y=250.0) -> (0:w840:bool)
                n259 = case shown="True" w840 {
                  tunnel: w839 -> [w854 w860]
                  tunnel: [w854 w859] -> w838
                  tunnel: [w847 w858] -> w837
                  tunnel: w836 -> [w846 w858]
                  frame False {
                    n260 = Unbundle(w846) -> ("D1"=w845:dbl, "D2"=w844:dbl, "D3"=w853:dbl, "D4"=w852:dbl, "D5"=w851:dbl, "D6"=w850:dbl, "D7"=w849:dbl, "D8"=w848:dbl)
                    n261 = Increment(x=w853) -> (x+1=w843:dbl)
                    n262 = Bundle("D1"=w845, "D2"=w844, w843, "D4"=w852, "D5"=w851, "D6"=w850, "D7"=w849, "D8"=w848) -> (w847:T9)  [unwired: 1 in]
                  }
                  frame True {
                    n263 = Unbundle(w860) -> ("D1"=w857:dbl, "D2"=w856:dbl, "D3"=w866:dbl, "D4"=w865:dbl, "D5"=w864:dbl, "D6"=w863:dbl, "D7"=w862:dbl, "D8"=w861:dbl)
                    n264 = Increment(x=w866) -> (x+1=w855:dbl)
                    n265 = Bundle("D1"=w857, "D2"=w856, w855, "D4"=w865, "D5"=w864, "D6"=w863, "D7"=w862, "D8"=w861) -> (w859:T9)  [unwired: 1 in]
                  }
                }
              }
              frame 3 {
                n266 = Greater?(x=w872, y=250.0) -> (0:w871:bool)
                n267 = case shown="True" w871 {
                  tunnel: w870 -> [w885 w892]
                  tunnel: [w885 w891] -> w869
                  tunnel: [w879 w890] -> w868
                  tunnel: w867 -> [w878 w890]
                  frame False {
                    n268 = Unbundle(w878) -> ("D1"=w877:dbl, "D2"=w876:dbl, "D3"=w875:dbl, "D4"=w884:dbl, "D5"=w883:dbl, "D6"=w882:dbl, "D7"=w881:dbl, "D8"=w880:dbl)
                    n269 = Increment(x=w884) -> (x+1=w874:dbl)
                    n270 = Bundle("D1"=w877, "D2"=w876, "D3"=w875, w874, "D5"=w883, "D6"=w882, "D7"=w881, "D8"=w880) -> (w879:T10)  [unwired: 1 in]
                  }
                  frame True {
                    n271 = Unbundle(w892) -> ("D1"=w889:dbl, "D2"=w888:dbl, "D3"=w887:dbl, "D4"=w897:dbl, "D5"=w896:dbl, "D6"=w895:dbl, "D7"=w894:dbl, "D8"=w893:dbl)
                    n272 = Increment(x=w897) -> (x+1=w886:dbl)
                    n273 = Bundle("D1"=w889, "D2"=w888, "D3"=w887, w886, "D5"=w896, "D6"=w895, "D7"=w894, "D8"=w893) -> (w891:T10)  [unwired: 1 in]
                  }
                }
              }
              frame 4 {
                n274 = Greater?(x=w903, y=250.0) -> (0:w902:bool)
                n275 = case shown="True" w902 {
                  tunnel: w901 -> [w916 w924]
                  tunnel: [w916 w923] -> w900
                  tunnel: [w911 w922] -> w899
                  tunnel: w898 -> [w910 w922]
                  frame False {
                    n276 = Unbundle(w910) -> ("D1"=w909:dbl, "D2"=w908:dbl, "D3"=w907:dbl, "D4"=w906:dbl, "D5"=w915:dbl, "D6"=w914:dbl, "D7"=w913:dbl, "D8"=w912:dbl)
                    n277 = Increment(x=w915) -> (x+1=w905:dbl)
                    n278 = Bundle("D1"=w909, "D2"=w908, "D3"=w907, "D4"=w906, w905, "D6"=w914, "D7"=w913, "D8"=w912) -> (w911:T11)  [unwired: 1 in]
                  }
                  frame True {
                    n279 = Unbundle(w924) -> ("D1"=w921:dbl, "D2"=w920:dbl, "D3"=w919:dbl, "D4"=w918:dbl, "D5"=w928:dbl, "D6"=w927:dbl, "D7"=w926:dbl, "D8"=w925:dbl)
                    n280 = Increment(x=w928) -> (x+1=w917:dbl)
                    n281 = Bundle("D1"=w921, "D2"=w920, "D3"=w919, "D4"=w918, w917, "D6"=w927, "D7"=w926, "D8"=w925) -> (w923:T11)  [unwired: 1 in]
                  }
                }
              }
              frame 5 {
                n282 = Greater?(x=w934, y=250.0) -> (0:w933:bool)
                n283 = case shown="True" w933 {
                  tunnel: w932 -> [w947 w956]
                  tunnel: [w947 w955] -> w931
                  tunnel: [w943 w954] -> w930
                  tunnel: w929 -> [w942 w954]
                  frame False {
                    n284 = Unbundle(w942) -> ("D1"=w941:dbl, "D2"=w940:dbl, "D3"=w939:dbl, "D4"=w938:dbl, "D5"=w937:dbl, "D6"=w946:dbl, "D7"=w945:dbl, "D8"=w944:dbl)
                    n285 = Increment(x=w946) -> (x+1=w936:dbl)
                    n286 = Bundle("D1"=w941, "D2"=w940, "D3"=w939, "D4"=w938, "D5"=w937, w936, "D7"=w945, "D8"=w944) -> (w943:T12)  [unwired: 1 in]
                  }
                  frame True {
                    n287 = Unbundle(w956) -> ("D1"=w953:dbl, "D2"=w952:dbl, "D3"=w951:dbl, "D4"=w950:dbl, "D5"=w949:dbl, "D6"=w959:dbl, "D7"=w958:dbl, "D8"=w957:dbl)
                    n288 = Increment(x=w959) -> (x+1=w948:dbl)
                    n289 = Bundle("D1"=w953, "D2"=w952, "D3"=w951, "D4"=w950, "D5"=w949, w948, "D7"=w958, "D8"=w957) -> (w955:T12)  [unwired: 1 in]
                  }
                }
              }
              frame 6 {
                n290 = Greater?(x=w965, y=250.0) -> (0:w964:bool)
                n291 = case shown="True" w964 {
                  tunnel: w963 -> [w978 w988]
                  tunnel: [w978 w987] -> w962
                  tunnel: [w975 w986] -> w961
                  tunnel: w960 -> [w974 w986]
                  frame False {
                    n292 = Unbundle(w974) -> ("D1"=w973:dbl, "D2"=w972:dbl, "D3"=w971:dbl, "D4"=w970:dbl, "D5"=w969:dbl, "D6"=w968:dbl, "D7"=w977:dbl, "D8"=w976:dbl)
                    n293 = Increment(x=w977) -> (x+1=w967:dbl)
                    n294 = Bundle("D1"=w973, "D2"=w972, "D3"=w971, "D4"=w970, "D5"=w969, "D6"=w968, w967, "D8"=w976) -> (w975:T13)  [unwired: 1 in]
                  }
                  frame True {
                    n295 = Unbundle(w988) -> ("D1"=w985:dbl, "D2"=w984:dbl, "D3"=w983:dbl, "D4"=w982:dbl, "D5"=w981:dbl, "D6"=w980:dbl, "D7"=w990:dbl, "D8"=w989:dbl)
                    n296 = Increment(x=w990) -> (x+1=w979:dbl)
                    n297 = Bundle("D1"=w985, "D2"=w984, "D3"=w983, "D4"=w982, "D5"=w981, "D6"=w980, w979, "D8"=w989) -> (w987:T13)  [unwired: 1 in]
                  }
                }
              }
              frame 7 {
                n298 = Greater?(x=w996, y=250.0) -> (0:w995:bool)
                n299 = case shown="True" w995 {
                  tunnel: w994 -> [w1009 w1020]
                  tunnel: [w1009 w1019] -> w993
                  tunnel: [w1007 w1018] -> w992
                  tunnel: w991 -> [w1006 w1018]
                  frame False {
                    n300 = Unbundle(w1006) -> ("D1"=w1005:dbl, "D2"=w1004:dbl, "D3"=w1003:dbl, "D4"=w1002:dbl, "D5"=w1001:dbl, "D6"=w1000:dbl, "D7"=w999:dbl, "D8"=w1008:dbl)
                    n301 = Increment(x=w1008) -> (x+1=w998:dbl)
                    n302 = Bundle("D1"=w1005, "D2"=w1004, "D3"=w1003, "D4"=w1002, "D5"=w1001, "D6"=w1000, "D7"=w999, w998) -> (w1007:T14)  [unwired: 1 in]
                  }
                  frame True {
                    n303 = Unbundle(w1020) -> ("D1"=w1017:dbl, "D2"=w1016:dbl, "D3"=w1015:dbl, "D4"=w1014:dbl, "D5"=w1013:dbl, "D6"=w1012:dbl, "D7"=w1011:dbl, "D8"=w1021:dbl)
                    n304 = Increment(x=w1021) -> (x+1=w1010:dbl)
                    n305 = Bundle("D1"=w1017, "D2"=w1016, "D3"=w1015, "D4"=w1014, "D5"=w1013, "D6"=w1012, "D7"=w1011, w1010) -> (w1019:T14)  [unwired: 1 in]
                  }
                }
              }
            }
          }
        }
      }
    }
  }
  "Object on 8 directions" <- w94
  "Enemy on 8 directions" <- w92
  "Closest valid target" <- w89
  n306 = Unbundle(w81) -> ("D1"=w58:dbl, "D2"=w57:dbl, "D3"=w56:dbl, "D4"=w55:dbl, "D5"=w54:dbl, "D6"=w53:dbl, "D7"=w52:dbl, "D8"=w51:dbl)
  n307 = Unbundle(w80) -> ("D1"=w17:dbl, "D2"=w16:dbl, "D3"=w15:dbl, "D4"=w14:dbl, "D5"=w13:dbl, "D6"=w12:dbl, "D7"=w11:dbl, "D8"=w10:dbl)
  n308 = Greater?(x=w54, y=2.0) -> (0:w70:bool)
  n309 = Greater?(x=w51, y=2.0) -> (0:w61:bool)
  n310 = Greater?(x=w55, y=2.0) -> (0:w73:bool)
  n311 = Greater?(x=w53, y=2.0) -> (0:w67:bool)
  n312 = Greater?(x=w52, y=2.0) -> (0:w64:bool)
  n313 = Greater?(x=w56, y=2.0) -> (0:w76:bool)
  n314 = Greater?(x=w58, y=2.0) -> (0:w84:bool)
  n315 = Greater?(x=w57, y=2.0) -> (0:w79:bool)
  n316 = Greater?(x=w13, y=2.0) -> (0:w38:bool)
  n317 = Greater?(x=w10, y=2.0) -> (0:w29:bool)
  n318 = Greater?(x=w14, y=2.0) -> (0:w41:bool)
  n319 = Greater?(x=w12, y=2.0) -> (0:w35:bool)
  n320 = Greater?(x=w11, y=2.0) -> (0:w32:bool)
  n321 = Greater?(x=w15, y=2.0) -> (0:w44:bool)
  n322 = Greater?(x=w17, y=2.0) -> (0:w50:bool)
  n323 = Greater?(x=w16, y=2.0) -> (0:w47:bool)
  n324 = Select(t=2.0, s=w70, f=w54) -> (s? t:f=w22:dbl)
  n325 = Select(t=2.0, s=w61, f=w51) -> (s? t:f=w19:dbl)
  n326 = Select(t=2.0, s=w73, f=w55) -> (s? t:f=w23:dbl)
  n327 = Select(t=2.0, s=w67, f=w53) -> (s? t:f=w21:dbl)
  n328 = Select(t=2.0, s=w64, f=w52) -> (s? t:f=w20:dbl)
  n329 = Select(t=2.0, s=w76, f=w56) -> (s? t:f=w24:dbl)
  n330 = Select(t=2.0, s=w84, f=w58) -> (s? t:f=w26:dbl)
  n331 = Select(t=2.0, s=w79, f=w57) -> (s? t:f=w25:dbl)
  n332 = Select(t=2.0, s=w38, f=w13) -> (s? t:f=w5:dbl)
  n333 = Select(t=2.0, s=w29, f=w10) -> (s? t:f=w2:dbl)
  n334 = Select(t=2.0, s=w41, f=w14) -> (s? t:f=w6:dbl)
  n335 = Select(t=2.0, s=w35, f=w12) -> (s? t:f=w4:dbl)
  n336 = Select(t=2.0, s=w32, f=w11) -> (s? t:f=w3:dbl)
  n337 = Select(t=2.0, s=w44, f=w15) -> (s? t:f=w7:dbl)
  n338 = Select(t=2.0, s=w50, f=w17) -> (s? t:f=w9:dbl)
  n339 = Select(t=2.0, s=w47, f=w16) -> (s? t:f=w8:dbl)
  n340 = Bundle("D1"=w26, "D2"=w25, "D3"=w24, "D4"=w23, "D5"=w22, "D6"=w21, "D7"=w20, "D8"=w19) -> (→"Closer Bullets on 8 directions":T3)  [unwired: 1 in]
  n341 = Bundle("D1"=w9, "D2"=w8, "D3"=w7, "D4"=w6, "D5"=w5, "D6"=w4, "D7"=w3, "D8"=w2) -> (→"Farther Bullets on 8 directions":T3)  [unwired: 1 in]
